vi "MFR - Complete.vi"(0 "Flow, SPL & Audio":dynamicdata(graph), 9 "File Name In":path, 11 "Error In":errorcluster) -> (4 "Mean Flow (Overall)":dbl format="%0.3f", 6 "SPL Array":dbl[](array[numeric]), 8 "F0 Array":dbl[](array[numeric]), 10 "File Name":path, 15 "Error Out":errorcluster)   [LabVIEW 2020]
uses:
  <vilib>/Utility/miscctls.llb/LVCursorListTypeDef.ctl
  <vilib>/Analysis/baseanly.llb/Mean (DBL).vi
  <vilib>/Waveform/WDTOps.llb/WDT Get Waveform Subset DBL.vi
  <vilib>/Waveform/WDTOps.llb/WDT Get XY Value DBL.vi
  <vilib>/Analysis/NI_AALBase.lvlib
panel:
  out "F0 (Section)":dbl
  in  "Undo Button":bool
  out "Mean SPL":dbl format="%0.3f"
  out "Sections Marked":i32
  in  "Mark MFR":bool
  out "Mean Flow (Section)":dbl format="%0.3f"
  out "End Flow":dbl format="%0.3f"
  out "Start Flow":dbl format="%0.3f"
  out "Subset":dynamicdata(graph)
  out "Full":dynamicdata(graph)
  in  "OK":bool
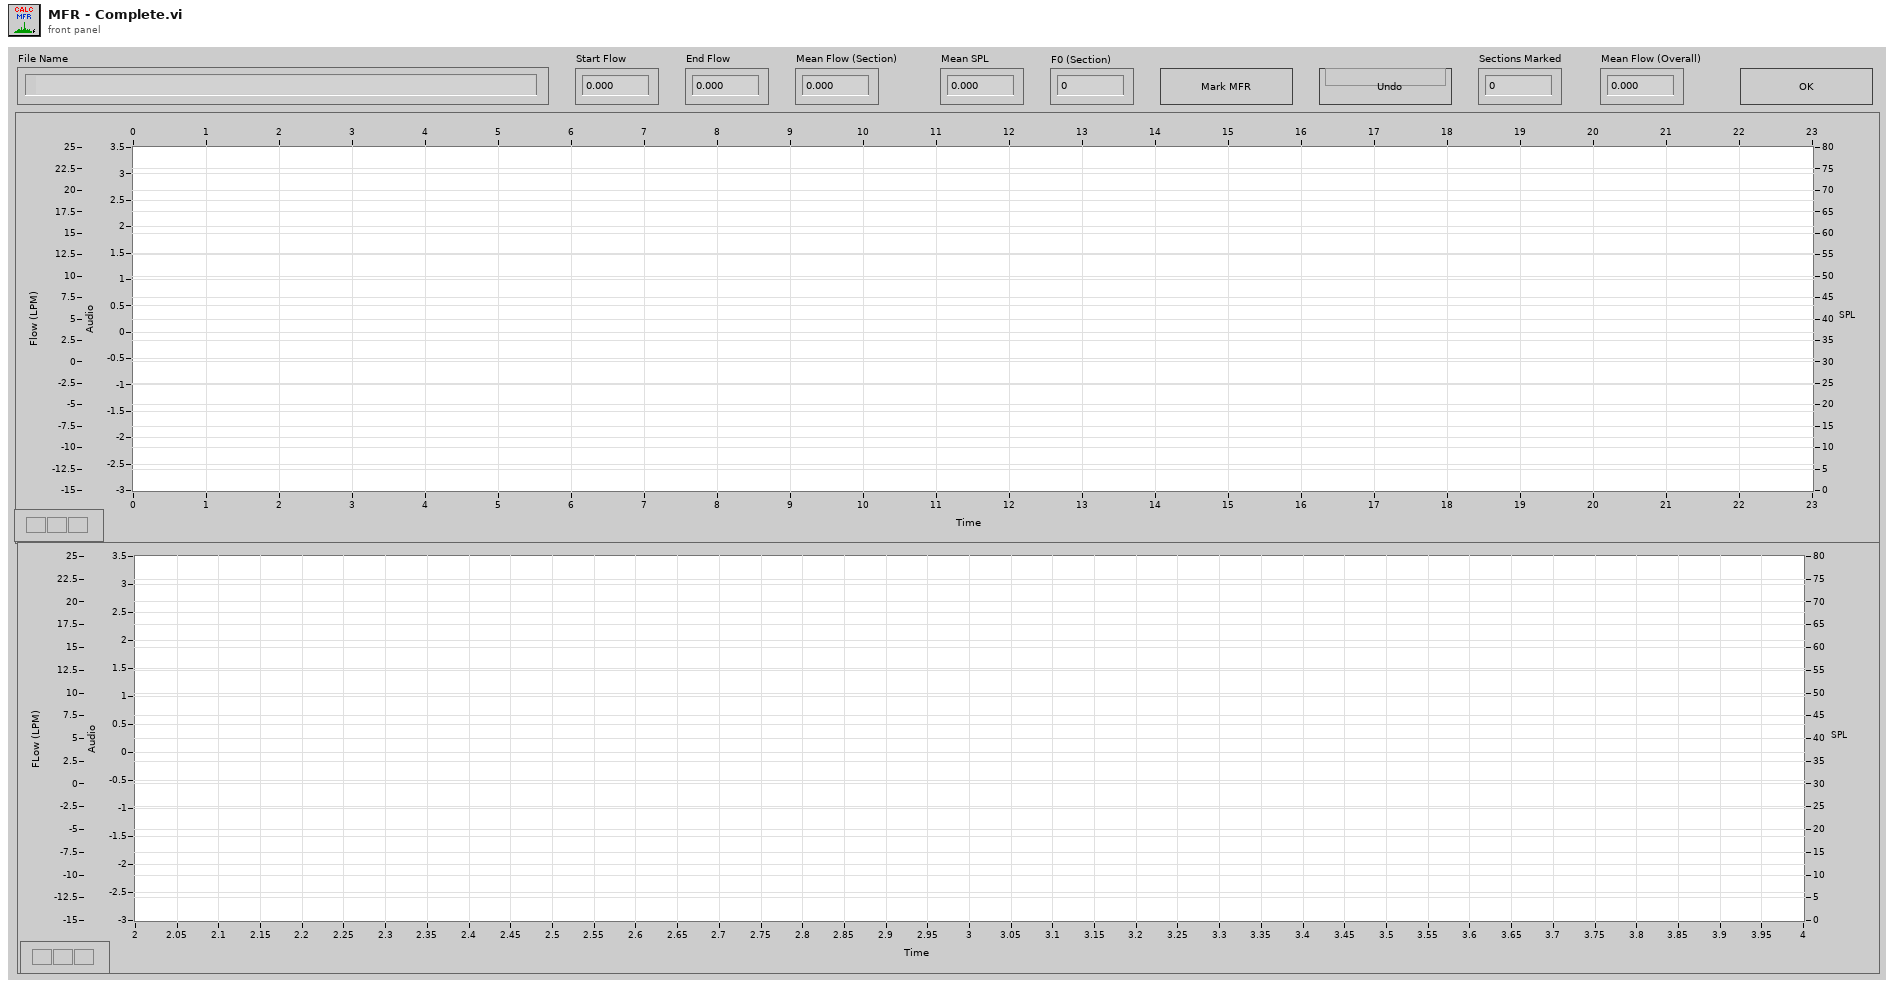
[diagram p1: front panel]
types:
  T1 = typedef "LVCursorListTypeDef.ctl" = cluster{"Name":string, "Color":u32, "Style":u8, "Point Style":u8, "Name Visible":bool, "Allow Drag":bool, "Cursor Mode":u32, "Plot":i32, "Index":i32, "Position":cluster{"X":dbl, "Y":dbl}, "X Scale":u32, "Y Scale":u32, "Watch Plots":i32[], "Watch All Plots":bool, "Plot Area":i32, "Label Offset":cluster{"X":dbl, "Y":dbl}}[]
  T2 = cluster{"Cursor List[0]":cluster{"Name":string, "Color":u32, "Style":u8, "Point Style":u8, "Name Visible":bool, "Allow Drag":bool, "Cursor Mode":u32, "Plot":i32, "Index":i32, "Position":cluster{"X":dbl, "Y":dbl}, "X Scale":u32, "Y Scale":u32, "Watch Plots":i32[], "Watch All Plots":bool, "Plot Area":i32, "Label Offset":cluster{"X":dbl, "Y":dbl}}, "Cursor List[1]":cluster{"Name":string, "Color":u32, "Style":u8, "Point Style":u8, "Name Visible":bool, "Allow Drag":bool, "Cursor Mode":u32, "Plot":i32, "Index":i32, "Position":cluster{"X":dbl, "Y":dbl}, "X Scale":u32, "Y Scale":u32, "Watch Plots":i32[], "Watch All Plots":bool, "Plot Area":i32, "Label Offset":cluster{"X":dbl, "Y":dbl}}, "Cursor List[2]":cluster{"Name":string, "Color":u32, "Style":u8, "Point Style":u8, "Name Visible":bool, "Allow Drag":bool, "Cursor Mode":u32, "Plot":i32, "Index":i32, "Position":cluster{"X":dbl, "Y":dbl}, "X Scale":u32, "Y Scale":u32, "Watch Plots":i32[], "Watch All Plots":bool, "Plot Area":i32, "Label Offset":cluster{"X":dbl, "Y":dbl}}, "Cursor List[3]":cluster{"Name":string, "Color":u32, "Style":u8, "Point Style":u8, "Name Visible":bool, "Allow Drag":bool, "Cursor Mode":u32, "Plot":i32, "Index":i32, "Position":cluster{"X":dbl, "Y":dbl}, "X Scale":u32, "Y Scale":u32, "Watch Plots":i32[], "Watch All Plots":bool, "Plot Area":i32, "Label Offset":cluster{"X":dbl, "Y":dbl}}, "Cursor List[4]":cluster{"Name":string, "Color":u32, "Style":u8, "Point Style":u8, "Name Visible":bool, "Allow Drag":bool, "Cursor Mode":u32, "Plot":i32, "Index":i32, "Position":cluster{"X":dbl, "Y":dbl}, "X Scale":u32, "Y Scale":u32, "Watch Plots":i32[], "Watch All Plots":bool, "Plot Area":i32, "Label Offset":cluster{"X":dbl, "Y":dbl}}, "Cursor List[5]":cluster{"Name":string, "Color":u32, "Style":u8, "Point Style":u8, "Name Visible":bool, "Allow Drag":bool, "Cursor Mode":u32, "Plot":i32, "Index":i32, "Position":cluster{"X":dbl, "Y":dbl}, "X Scale":u32, "Y Scale":u32, "Watch Plots":i32[], "Watch All Plots":bool, "Plot Area":i32, "Label Offset":cluster{"X":dbl, "Y":dbl}}, "Cursor List[6]":cluster{"Name":string, "Color":u32, "Style":u8, "Point Style":u8, "Name Visible":bool, "Allow Drag":bool, "Cursor Mode":u32, "Plot":i32, "Index":i32, "Position":cluster{"X":dbl, "Y":dbl}, "X Scale":u32, "Y Scale":u32, "Watch Plots":i32[], "Watch All Plots":bool, "Plot Area":i32, "Label Offset":cluster{"X":dbl, "Y":dbl}}, "Cursor List[7]":cluster{"Name":string, "Color":u32, "Style":u8, "Point Style":u8, "Name Visible":bool, "Allow Drag":bool, "Cursor Mode":u32, "Plot":i32, "Index":i32, "Position":cluster{"X":dbl, "Y":dbl}, "X Scale":u32, "Y Scale":u32, "Watch Plots":i32[], "Watch All Plots":bool, "Plot Area":i32, "Label Offset":cluster{"X":dbl, "Y":dbl}}, "Cursor List[8]":cluster{"Name":string, "Color":u32, "Style":u8, "Point Style":u8, "Name Visible":bool, "Allow Drag":bool, "Cursor Mode":u32, "Plot":i32, "Index":i32, "Position":cluster{"X":dbl, "Y":dbl}, "X Scale":u32, "Y Scale":u32, "Watch Plots":i32[], "Watch All Plots":bool, "Plot Area":i32, "Label Offset":cluster{"X":dbl, "Y":dbl}}}
  T3 = cluster{"Name":string, "Color":u32, "Style":u8, "Point Style":u8, "Name Visible":bool, "Allow Drag":bool, "Cursor Mode":u32, "Plot":i32, "Index":i32, "Position":cluster{"X":dbl, "Y":dbl}, "X Scale":u32, "Y Scale":u32, "Watch Plots":i32[], "Watch All Plots":bool, "Plot Area":i32, "Label Offset":cluster{"X":dbl, "Y":dbl}}[]
  T4 = cluster{"CrsrList[0]":cluster{"Name":string, "Color":u32, "Style":u8, "Point Style":u8, "Name Visible":bool, "Allow Drag":bool, "Cursor Mode":u32, "Plot":i32, "Index":i32, "Position":cluster{"X":dbl, "Y":dbl}, "X Scale":u32, "Y Scale":u32, "Watch Plots":i32[], "Watch All Plots":bool, "Plot Area":i32, "Label Offset":cluster{"X":dbl, "Y":dbl}}, "CrsrList[1]":cluster{"Name":string, "Color":u32, "Style":u8, "Point Style":u8, "Name Visible":bool, "Allow Drag":bool, "Cursor Mode":u32, "Plot":i32, "Index":i32, "Position":cluster{"X":dbl, "Y":dbl}, "X Scale":u32, "Y Scale":u32, "Watch Plots":i32[], "Watch All Plots":bool, "Plot Area":i32, "Label Offset":cluster{"X":dbl, "Y":dbl}}, "CrsrList[2]":cluster{"Name":string, "Color":u32, "Style":u8, "Point Style":u8, "Name Visible":bool, "Allow Drag":bool, "Cursor Mode":u32, "Plot":i32, "Index":i32, "Position":cluster{"X":dbl, "Y":dbl}, "X Scale":u32, "Y Scale":u32, "Watch Plots":i32[], "Watch All Plots":bool, "Plot Area":i32, "Label Offset":cluster{"X":dbl, "Y":dbl}}, "CrsrList[3]":cluster{"Name":string, "Color":u32, "Style":u8, "Point Style":u8, "Name Visible":bool, "Allow Drag":bool, "Cursor Mode":u32, "Plot":i32, "Index":i32, "Position":cluster{"X":dbl, "Y":dbl}, "X Scale":u32, "Y Scale":u32, "Watch Plots":i32[], "Watch All Plots":bool, "Plot Area":i32, "Label Offset":cluster{"X":dbl, "Y":dbl}}, "CrsrList[4]":cluster{"Name":string, "Color":u32, "Style":u8, "Point Style":u8, "Name Visible":bool, "Allow Drag":bool, "Cursor Mode":u32, "Plot":i32, "Index":i32, "Position":cluster{"X":dbl, "Y":dbl}, "X Scale":u32, "Y Scale":u32, "Watch Plots":i32[], "Watch All Plots":bool, "Plot Area":i32, "Label Offset":cluster{"X":dbl, "Y":dbl}}, "CrsrList[5]":cluster{"Name":string, "Color":u32, "Style":u8, "Point Style":u8, "Name Visible":bool, "Allow Drag":bool, "Cursor Mode":u32, "Plot":i32, "Index":i32, "Position":cluster{"X":dbl, "Y":dbl}, "X Scale":u32, "Y Scale":u32, "Watch Plots":i32[], "Watch All Plots":bool, "Plot Area":i32, "Label Offset":cluster{"X":dbl, "Y":dbl}}, "CrsrList[6]":cluster{"Name":string, "Color":u32, "Style":u8, "Point Style":u8, "Name Visible":bool, "Allow Drag":bool, "Cursor Mode":u32, "Plot":i32, "Index":i32, "Position":cluster{"X":dbl, "Y":dbl}, "X Scale":u32, "Y Scale":u32, "Watch Plots":i32[], "Watch All Plots":bool, "Plot Area":i32, "Label Offset":cluster{"X":dbl, "Y":dbl}}, "CrsrList[7]":cluster{"Name":string, "Color":u32, "Style":u8, "Point Style":u8, "Name Visible":bool, "Allow Drag":bool, "Cursor Mode":u32, "Plot":i32, "Index":i32, "Position":cluster{"X":dbl, "Y":dbl}, "X Scale":u32, "Y Scale":u32, "Watch Plots":i32[], "Watch All Plots":bool, "Plot Area":i32, "Label Offset":cluster{"X":dbl, "Y":dbl}}, "CrsrList[8]":cluster{"Name":string, "Color":u32, "Style":u8, "Point Style":u8, "Name Visible":bool, "Allow Drag":bool, "Cursor Mode":u32, "Plot":i32, "Index":i32, "Position":cluster{"X":dbl, "Y":dbl}, "X Scale":u32, "Y Scale":u32, "Watch Plots":i32[], "Watch All Plots":bool, "Plot Area":i32, "Label Offset":cluster{"X":dbl, "Y":dbl}}}
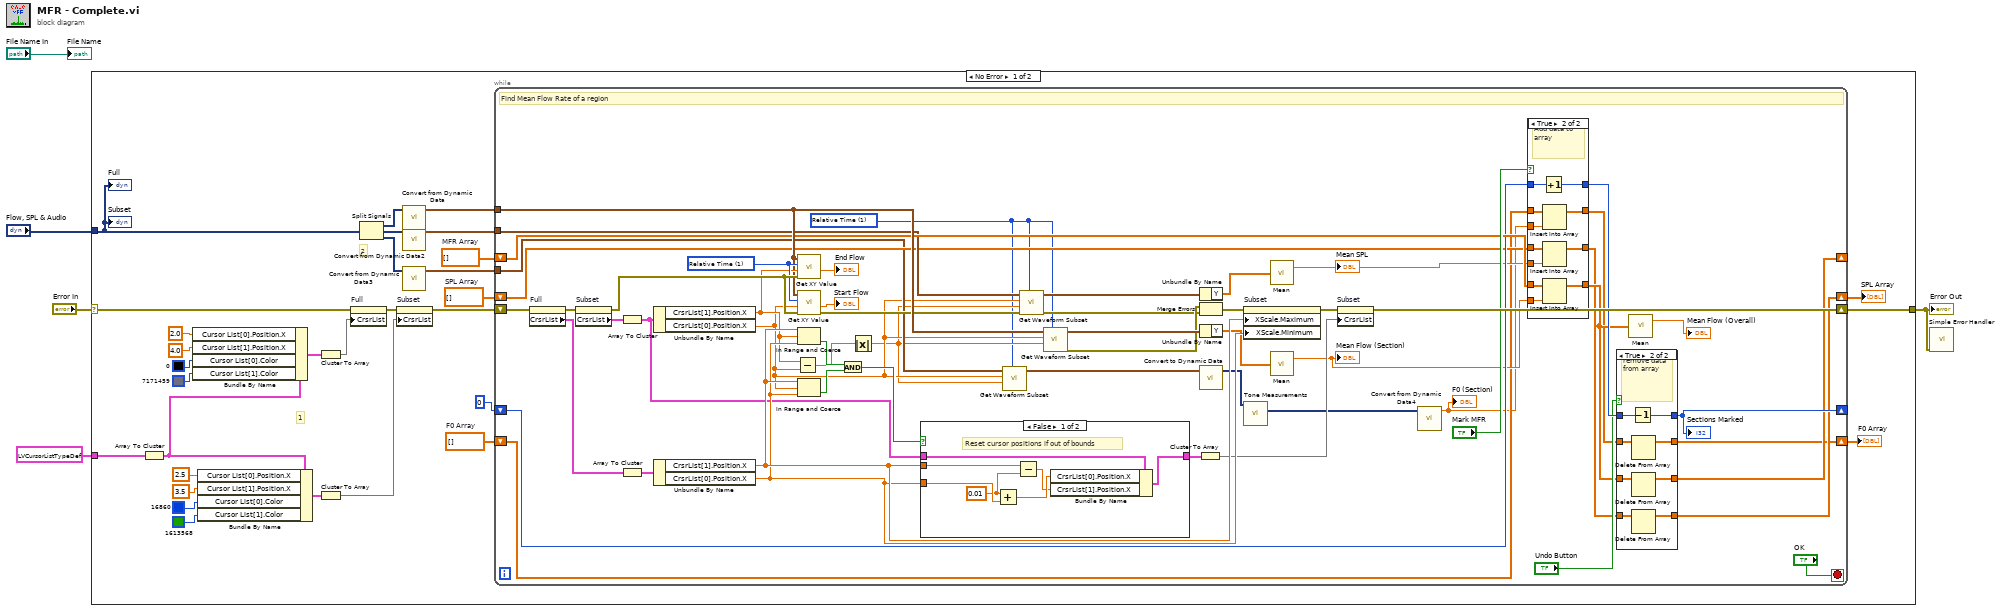
[diagram p0: block diagram]
diagram:
  n1 = case shown="No Error" "Error In" {
    selector: "Error In" -> [w11 w129]
    tunnel: "Flow, SPL & Audio" -> [w15 _]
    tunnel: [w36 w129] -> w1
    tunnel: T1 [{"Name"="Left", "Color"=9843450, "Style"=2, "Point Style"=1, "Name Visible"=FALSE, "Allow Drag"=TRUE, "Cursor Mode"=0, "Plot"=0, "Index"=0, "Position"={"X"=3.0, "Y"=0.0}, "X Scale"=0, "Y Scale"=0, "Watch Plots"=[], "Watch All Plots"=FALSE, "Plot Area"=0, "Label Offset"={"X"=0.0, "Y"=0.0}}, {"Name"="Right", "Color"=681210, "Style"=2, "Point Style"=1, "Name Visible"=FALSE, "Allow Drag"=TRUE, "Cursor Mode"=0, "Plot"=0, "Index"=0, "Position"={"X"=3.5, "Y"=0.0}, "X Scale"=0, "Y Scale"=0, "Watch Plots"=[], "Watch All Plots"=FALSE, "Plot Area"=0, "Label Offset"={"X"=0.0, "Y"=0.0}}, {"Name"="Middle", "Color"=4617539, "Style"=2, "Point Style"=1, "Name Visible"=FALSE, "Allow Drag"=TRUE, "Cursor Mode"=0, "Plot"=0, "Index"=0, "Position"={"X"=0.0, "Y"=0.0}, "X Scale"=0, "Y Scale"=0, "Watch Plots"=[], "Watch All Plots"=FALSE, "Plot Area"=0, "Label Offset"={"X"=0.0, "Y"=0.0}}] ("Cursor List") -> [w34 _]
    frame No Error {
      w7 = dbl[] []  # F0 Array
      w12 = dbl[] []  # SPL Array
      w18 = dbl[] []  # MFR Array
      # "2"
      # "1"
      n2 = Array To Cluster(array=w34) -> (cluster=w28:T2)
      n3 = Bundle By Name(cluster=w28, "Cursor List[0].Position.X"=2.0, "Cursor List[1].Position.X"=4.0, "Cursor List[0].Color"=u32 0, "Cursor List[1].Color"=u32 7171459) -> (w32:T2)
      n4 = Bundle By Name(cluster=w28, "Cursor List[0].Position.X"=2.5, "Cursor List[1].Position.X"=3.5 ("Cursor List[0].Position.Y"), "Cursor List[0].Color"=u32 16860, "Cursor List[1].Color"=u32 1613568) -> (w30:T2)
      n5 = Cluster To Array(cluster=w32) -> (array=w31:T3)
      n6 = Cluster To Array(cluster=w30) -> (array=w29:T3)
      n7 = property on="Full" class="WFGraph (strict)"(error in=w11, "CrsrList"=w31) -> (error out=w33:errorcluster)  [unwired: 1 in, 1 out]
      n8 = Split Signals(w15) -> (w16:dynamicdata, w14:dynamicdata, w9:dynamicdata)  [unwired: 3 in]
      n9 = property on="Subset" class="WFGraph (strict)"(error in=w33, "CrsrList"=w29) -> (error out=w27:errorcluster)  [unwired: 1 in, 1 out]
      n10 = call "Convert from Dynamic Data"("Dynamic Data Type"=w16) -> ("Waveform"=w35:waveform(dbl))  [unwired: 3 in]
      n11 = call "Convert from Dynamic Data2"("Dynamic Data Type"=w14) -> ("Waveform"=w13:waveform(dbl))  [unwired: 3 in]
      n12 = call "Convert from Dynamic Data3"("Dynamic Data Type"=w9) -> ("Waveform"=w8:waveform(dbl))  [unwired: 3 in]
      n13 = while {
        shift-right: [w82] -> w36
        shift-left: w27 -> [w85]
        tunnel: w35 -> [w70]
        shift-right: [w50] -> _
        shift-left: w18 -> [w67]
        tunnel: w13 -> [w58]
        shift-right: [w48] -> w10
        shift-left: w12 -> [w56]
        shift-right: [w53] -> _
        shift-left: 0 -> [w66]
        tunnel: w8 -> [w47]
        shift-right: [w37] -> w6
        shift-left: w7 -> [w41]
        stop <- "OK" stop-if-true
        w42 = u16 1 items=["Samples", "Relative Time"] ("start/duration format")
        w78 = u16 1 items=["Samples", "Relative Time"] ("start/duration format")
        # "Find Mean Flow Rate of a region"
        n14 = property on="Full" class="WFGraph (strict)"(error in=w85) -> (error out=w71:errorcluster, "CrsrList"=w83:T1)  [unwired: 1 in, 1 out]
        n15 = property on="Subset" class="WFGraph (strict)"(error in=w71) -> (error out=w80:errorcluster, "CrsrList"=w76:T1)  [unwired: 1 in, 1 out]
        n16 = Array To Cluster(array=w76) -> (cluster=w74:T4)
        n17 = Array To Cluster(array=w83) -> (cluster=w92:T4)
        n18 = Unbundle By Name(w74) -> ("CrsrList[1].Position.X"=w75:dbl, "CrsrList[0].Position.X"=w46:dbl)
        n19 = Unbundle By Name(w92) -> ("CrsrList[1].Position.X"=w91:dbl, "CrsrList[0].Position.X"=w90:dbl)
        n20 = Subtract(x=w75, y=w46) -> (x-y=w86:dbl)
        n21 = call-poly <vilib>:"Get XY Value.vi"("error in (no error)"=w80, "Y position"=w75, "Y position format"=w78, "waveform in"=w70) -> ("Y value"=→"End Flow":dbl)  [unwired: 3 in, 4 out]
        n22 = call-poly <vilib>:"Get XY Value.vi"("error in (no error)"=w80, "Y position"=w46, "Y position format"=w78, "waveform in"=w70) -> ("error out"=w59:errorcluster, "Y value"=→"Start Flow":dbl)  [unwired: 3 in, 3 out]
        n23 = In Range and Coerce(upper limit=w91, x=w75, lower limit=w90) -> (In Range?=w89:bool)  [unwired: 1 out]
        n24 = In Range and Coerce(upper limit=w91, x=w46, lower limit=w90) -> (In Range?=w88:bool)  [unwired: 1 out]
        n25 = And(x=w89, y=w88) -> (x .and. y?=w87:bool)
        n26 = Absolute Value(x=w86) -> (abs(x)=w45:dbl)
        n27 = case shown="False" w87 {
          tunnel: w91 -> [w127 _]
          tunnel: w90 -> [w126 _]
          tunnel: w74 -> [w124 w128]
          tunnel: [w123 w128] -> w73
          frame False {
            w125 = 0.01 ("y")
            # "Reset cursor positions if out of bounds"
            # "Right Cursor"
            n28 = Add(x=w125, y=w126) -> (x+y=w122:dbl)
            n29 = Subtract(x=w127, y=w125) -> (x-y=w121:dbl)
            n30 = Bundle By Name(cluster=w124, "CrsrList[0].Position.X"=w122, "CrsrList[1].Position.X"=w121) -> (w123:T4)
          }
          frame True {
            # "Right Cursor"
          }
        }
        n31 = call-poly <vilib>:"Get Waveform Subset.vi"("start/duration format"=w42, "duration"=w45, "start samples/time"=w46, "waveform in"=w47) -> ("waveform out"=w44:waveform(dbl))  [unwired: 2 in, 3 out]
        n32 = call-poly <vilib>:"Get Waveform Subset.vi"("start/duration format"=w42, "error in (no error)"=w59, "duration"=w45, "start samples/time"=w46, "waveform in"=w58) -> ("error out"=w61:errorcluster, "waveform out"=w57:waveform(dbl))  [unwired: 1 in, 2 out]
        n33 = call-poly <vilib>:"Get Waveform Subset.vi"("start/duration format"=w42, "duration"=w45, "start samples/time"=w46, "waveform in"=w70) -> ("error out"=w62:errorcluster, "waveform out"=w69:waveform(dbl))  [unwired: 2 in, 2 out]
        n34 = Cluster To Array(cluster=w73) -> (array=w77:T3)
        n35 = Unbundle By Name(w57) -> ("Y"=w60:dbl[])
        n36 = Merge Errors(w62, w61) -> (w63:errorcluster)
        n37 = Unbundle By Name(w69) -> ("Y"=w68:dbl[])
        n38 = call "Convert to Dynamic Data"("Waveform"=w44) -> ("Dynamic Data Type"=w43:dynamicdata)  [unwired: 3 in]
        n39 = property on="Subset" class="WFGraph (strict)"(error in=w63, "XScale.Maximum"=w91, "XScale.Minimum"=w90) -> (error out=w84:errorcluster)  [unwired: 1 in, 1 out]
        n40 = call "Tone Measurements"("Signals"=w43) -> ("Frequency"=w40:dynamicdata)  [unwired: 9 in, 1 out]
        n41 = call-poly <vilib>:"Mean.vi"("X"=w60) -> ("mean"=w55:dbl)  [unwired: 1 out]
        "Mean SPL" <- w55
        n42 = call-poly <vilib>:"Mean.vi"("X"=w68) -> ("mean"=w65:dbl)  [unwired: 1 out]
        "Mean Flow (Section)" <- w65
        n43 = property on="Subset" class="WFGraph (strict)"(error in=w84, "CrsrList"=w77) -> (error out=w82:errorcluster)  [unwired: 1 in, 1 out]
        n44 = call "Convert from Dynamic Data4"("Dynamic Data Type"=w40) -> ("Scalar"=w39:dbl)  [unwired: 3 in]
        "F0 (Section)" <- w39
        n45 = case shown="True" "Mark MFR" {
          tunnel: w67 -> [w108 w118]
          tunnel: [w109 w120] -> w54
          tunnel: w66 -> [w109 w119]
          tunnel: w65 -> [_ w117]
          tunnel: [w108 w116] -> w51
          tunnel: w56 -> [w107 w115]
          tunnel: w55 -> [_ w114]
          tunnel: [w107 w113] -> w49
          tunnel: w41 -> [w106 w112]
          tunnel: w39 -> [_ w111]
          tunnel: [w106 w110] -> w38
          frame False {
            # "Nothing"
          }
          frame True {
            # "Add data to array"
            n46 = Increment(x=w119) -> (x+1=w120:i32)
            n47 = Insert Into Array(array=w112, new element=w111) -> (w110:dbl[])  [unwired: 1 in]
            n48 = Insert Into Array(array=w115, new element=w114) -> (w113:dbl[])  [unwired: 1 in]
            n49 = Insert Into Array(array=w118, new element=w117) -> (w116:dbl[])  [unwired: 1 in]
          }
        }
        n50 = case shown="True" "Undo Button" {
          tunnel: w49 -> [w96 w104]
          tunnel: w54 -> [w97 w102]
          tunnel: [w97 w105] -> w53
          tunnel: [w96 w103] -> w48
          tunnel: w51 -> [w95 w101]
          tunnel: [w95 w100] -> w50
          tunnel: w38 -> [w94 w99]
          tunnel: [w94 w98] -> w37
          frame False {
            # "Nothing"
          }
          frame True {
            # "remove data from array"
            n51 = Decrement(x=w102) -> (x-1=w105:i32)
            n52 = Delete From Array(array=w99) -> (array with subset deleted=w98:dbl[])  [unwired: 2 in, 1 out]
            n53 = Delete From Array(array=w101) -> (array with subset deleted=w100:dbl[])  [unwired: 2 in, 1 out]
            n54 = Delete From Array(array=w104) -> (array with subset deleted=w103:dbl[])  [unwired: 2 in, 1 out]
          }
        }
        "Sections Marked" <- w53
        n55 = call-poly <vilib>:"Mean.vi"("X"=w51) -> ("mean"=→"Mean Flow (Overall)":dbl)  [unwired: 1 out]
      }
      "SPL Array" <- w10
      "F0 Array" <- w6
      "Full" <- w15
      "Subset" <- w15
    }
    frame Error {
    }
  }
  "Error Out" <- w1
  n56 = call <vilib>:"Simple Error Handler.vi"("error in (no error)"=w1) -> ()  [unwired: 4 in, 5 out]
  "File Name" <- "File Name In"
